vi "MAIN_TL_move_to_ROI.vi"(5 "queue ASI stage":refnum<queue>, 6 "XYGraph Refnum":refnum<vi>, 7 "queue piezo":refnum<queue>, 8 "error in":errorcluster, 9 "variant":variant, 10 "XY positions":dbl[][](array[numeric])) -> (0 "error out":errorcluster, 3 "Next task":T1)   [LabVIEW 2015]
uses:
  CONTROLS/Q_MCL_piezo_element.ctl
  CONTROLS/Q_ASI_stage_element.ctl
  CONTROLS/Q_main_element.ctl
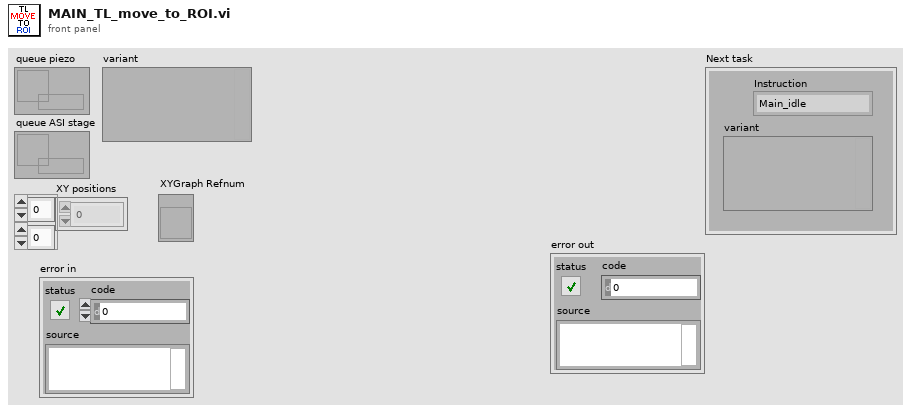
[diagram p1: front panel]
types:
  T1 = typedef "Q_main_element.ctl" = cluster{"variant":variant, "Instruction":enum16{"Main_idle", "Main_initialize", "Main_initialize_TDMS", "Main_initialize_Queue", "Main_error", "Main_DAQ_initialization_results", "Main_ASI_initialization_results", "Main_Piezo_initialization_results", "Main_Valve_initialization_results", "Main_Pump_initialization_results", "Main_CAMERA_initialization_results", "Main_DAQ_error", "Main_ASI_error", "Main_Piezo_error", "Main_CAMERA_error", "Main_Valve_error", "Main_Pump_error", "Main_start_acquiring", "Main_not_acquiring", "Main_acquiring", "Main_stop_acquiring", "Main_change_exposure", "Main_change_z_scan_parameters", "Main_define_ROI", "Main_define_mosaic", "Main_read_kinetic_time", "Main_cooler", "Main_read_temperature", "Main_save_XY", "Main_load_XY", "Main_discard_XY", "Main_move_to_XY", "Main_measure_QPD", "Main_autofocus_calibration", "Main_save_PID", "Main_change_H_valve_position", "Main_two_way_valve", "Main_save_movie", "Main_init_single_scan", "Main_single_scan", "Main_stop_single_scan", "Main_merFISH_illumination_parameters", "Main_merFISH_buffer_probe_list", "Main_merFISH_injections_procedure", "Main_merFISH_save_setpoint", "Main_merFISH_DAPI_parameters", "Main_merFISH_Brightfield_parameters", "Main_merFISH_save_embryo_ROI", "Main_merFISH_init", "Main_merFISH_resume", "Main_merFISH_start_autofocus", "Main_merFISH_open_close_valve_merFISH", "Main_merFISH_open_close_valve_photobleaching", "Main_merFISH_hybridization", "Main_merFISH_move_to_ROI", "Main_merFISH_wait_stabilization", "Main_merFISH_scan_laser", "Main_merFISH_scan_brightfield", "Main_merFISH_photobleaching_injection", "Main_merFISH_photobleaching", "Main_merFISH_save", "Main_merFISH_send_email", "Main_merFISH_close", "Main_TL_define_parameters", "Main_TL_reset_parameters", "Main_TL_init", "Main_TL_start_autofocus", "Main_TL_move_to_ROI", "Main_TL_wait_for_stabilization", "Main_TL_scan", "Main_TL_wait_cycle_end", "Main_TL_close", "Main_STOP"}}
  T2 = typedef "Q_ASI_stage_element.ctl" = cluster{"variant":variant, "Instruction":enum16{"ASI_idle", "ASI_initialize", "ASI_error", "ASI_security_stop", "ASI_read_XYZ", "ASI_up", "ASI_down", "ASI_left", "ASI_right", "ASI_save_XY", "ASI_move_to_XY", "ASI_brightfield", "ASI_init_scan", "ASI_init_merFISH", "ASI_move_to_XY_merFISH", "ASI_move_to_Z_merFISH", "ASI_init_autofocus_search_merFISH", "ASI_close_autofocus_search_merFISH", "ASI_adjust_piezo_autofocus_merFISH", "ASI_set_piezo_autofocus_to_reference_position_merFISH_TL", "ASI_close_merFISH", "ASI_init_TL", "ASI_move_mosaic_TL", "ASI_brightfield_TL", "ASI_close_TL", "ASI_stop"}}
  T3 = cluster{"XYGraph Refnum":refnum<vi>, "XY positions":dbl[]}
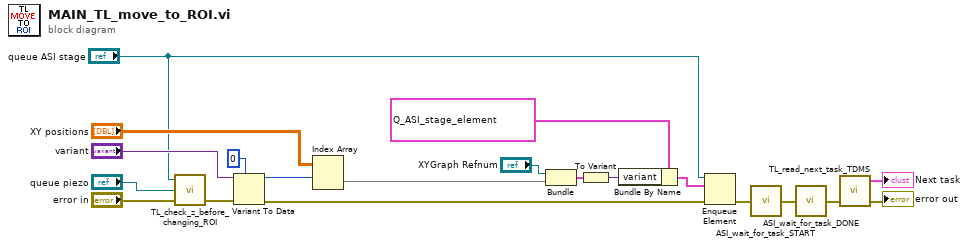
[diagram p0: block diagram]
diagram:
  n1 = call "TL_check_z_before_changing_ROI.vi"("error in"="error in", "queue piezo"="queue piezo", "queue ASI stage"="queue ASI stage") -> ("error out"=w10:errorcluster)  [unwired: 2 in]
  n2 = Variant To Data(error in=w10, type=0, Variant="variant") -> (data=w11:i32, error out=w13:errorcluster)
  n3 = Index Array(array="XY positions", index (row)=w11) -> (element=w12:dbl[])  [unwired: 1 in]
  n4 = Bundle("XYGraph Refnum"="XYGraph Refnum", "XY positions"=w12) -> (w15:T3)  [unwired: 1 in]
  n5 = To Variant(anything=w15) -> (Variant=w17:variant)
  n6 = Bundle By Name(cluster=T2 {"variant"=variant, "Instruction"=enum."ASI_move_mosaic_TL"} ("element"), "variant"=w17) -> (w18:T2)
  n7 = Enqueue Element(queue="queue ASI stage", element=w18, error in (no error)=w13) -> (error out=w14:errorcluster)  [unwired: 1 in, 2 out]
  n8 = call "ASI_wait_for_task_START.vi"("error in"=w14) -> ("error out"=w19:errorcluster)
  n9 = call "ASI_wait_for_task_DONE.vi"("error in"=w19) -> ("error out"=w20:errorcluster)
  n10 = call "TL_read_next_task_TDMS.vi"("error in"=w20) -> ("error out"=→"error out":errorcluster, "task"=→"Next task":T1)  [unwired: 3 in]
